vi "Goal Editor GUI.vi"(8 "error in (no error)":errorcluster, 10 "Cat Summary":refnum<class "Expense Summary.lvclass">, 11 "Database.lvclass":refnum<class "Database.lvclass">) -> (0 "error out":errorcluster, 3 "Database.lvclass":refnum<class "Database.lvclass">)   [LabVIEW 2018]
uses:
  support/classes/database/Database.lvclass
  support/classes/Expense Summary/Expense Summary.lvclass
panel:
  in  "Cancel":bool
  in  "Goal Amount":dbl
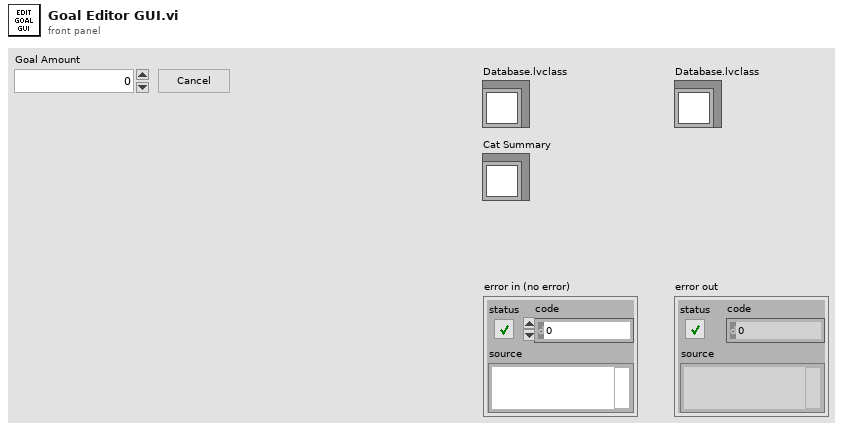
[diagram p1: front panel]
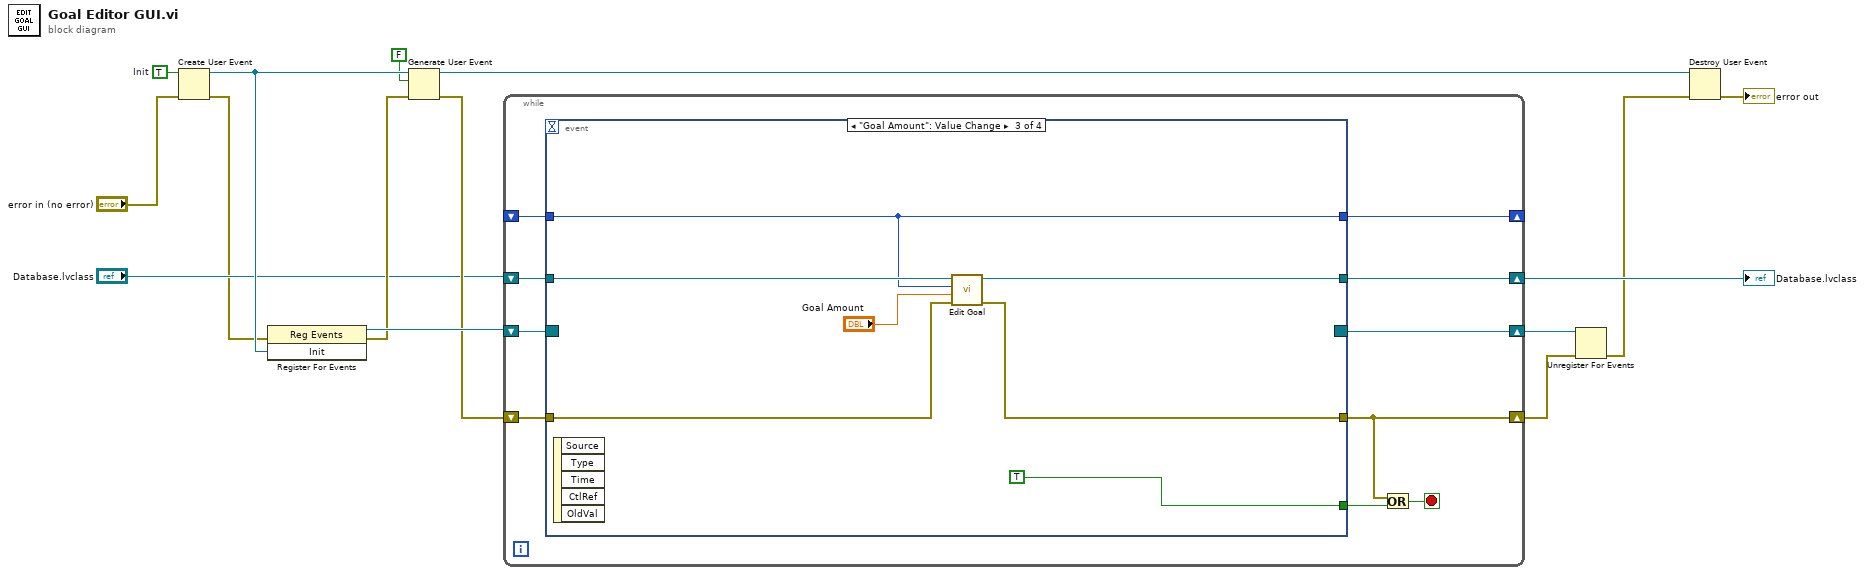
[diagram p0: block diagram]
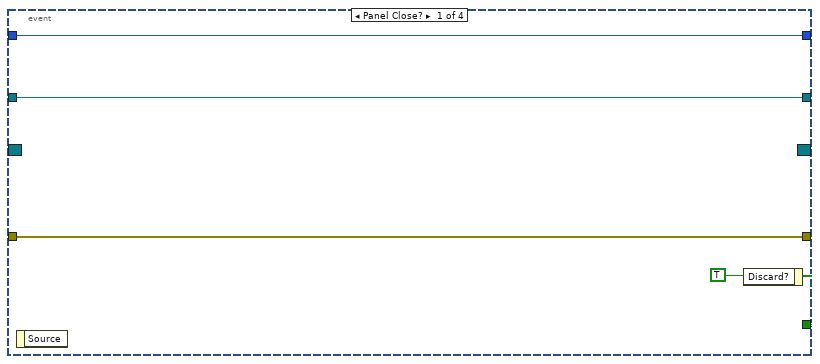
[diagram p2: hidden frame]
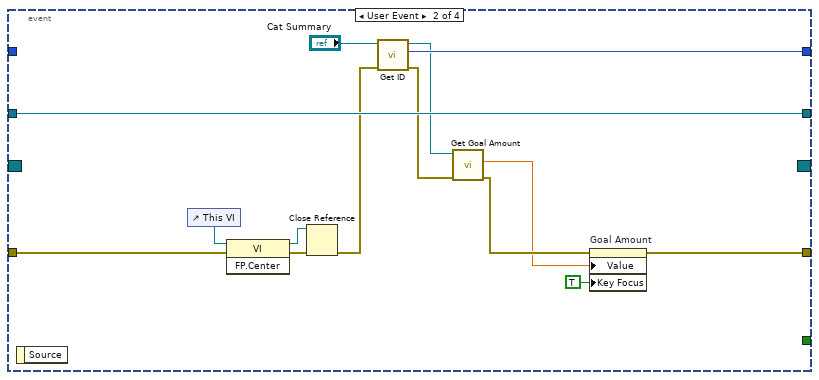
[diagram p3: hidden frame]
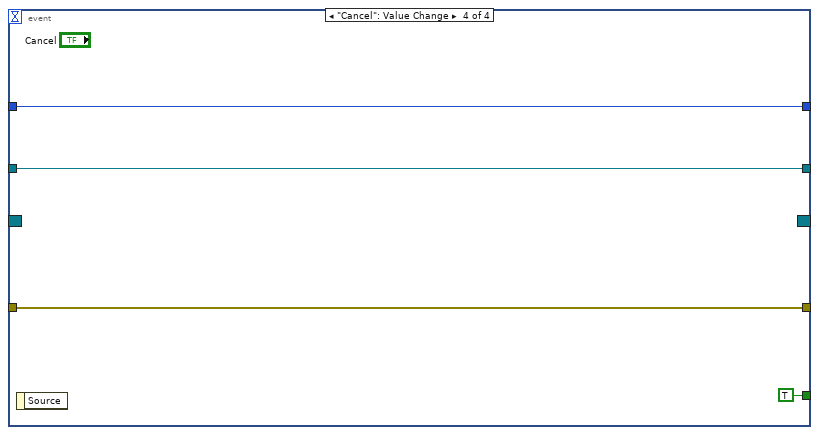
[diagram p4: hidden frame]
diagram:
  w15 = TRUE  # Init
  n1 = Create User Event(user event datatype=w15, error in="error in (no error)") -> (user event=w13:refnum<user-event>, error out=w7:errorcluster)
  n2 = register-events(error in=w7, w13) -> (reference out=w14:refnum<event-registration>, error out=w12:errorcluster)  [unwired: 1 in]
  n3 = Generate User Event(user event=w13, event data cluster=FALSE ("event data"), error in=w12) -> (user event out=w6:refnum<user-event>, error out=w11:errorcluster)  [unwired: 1 in]
  n4 = while {
    shift-right: [w23] -> w5
    shift-left: w14 -> [w25]
    shift-right: [w22] -> w4
    shift-left: w11 -> [w24]
    shift-right: [w18] -> w8
    shift-left: "Database.lvclass" -> [w19]
    shift-right: [w17] -> _
    shift-left: _ -> [w16]
    stop <- w20 stop-if-true
    n5 = event shown="[2] \"Goal Amount\": Value Change" {
      selector: w25 -> [_ _ _ _]
      dyn-events: [_ _ _ _] -> w23
      timeout: _ -> [_ _ _ _]
      tunnel: [w29 _ TRUE ("Discard?") TRUE ("Discard?")] -> w21
      tunnel: w24 -> [w28 w42 w47 w52]
      tunnel: [w28 w33 w48 w52] -> w22
      tunnel: w19 -> [w27 w39 w50 w53]
      tunnel: [w27 w39 w49 w53] -> w18
      tunnel: [w26 w37 w46 w51] -> w17
      tunnel: w16 -> [w26 _ w46 w51]
      event Panel Close? {
        w29 = TRUE ("Discard?")
        n6 = event-data() -> ()  [unwired: 1 in, 1 out]
        n7 = event-data("Discard?"=w29) -> ()  [unwired: 1 in, 1 out]
      }
      event User Event {
        n8 = event-data() -> ()  [unwired: 1 in, 1 out]
        n9 = control-ref of="This VI"() -> (w43:refnum<vi>)
        n10 = invoke class="VI" method="FP.Center"(reference=w43, error in=w42) -> (reference out=w40:refnum<vi>, error out=w41:errorcluster)  [unwired: 1 in, 1 out]
        n11 = Close Reference(reference=w40, error in (no error)=w41) -> (error out=w36:errorcluster)
        n12 = call "Get ID.vi"("error in (no error)"=w36, "Expense Summary in"="Cat Summary") -> ("error out"=w31:errorcluster, "goal_id"=w37:i32, "Expense Summary out"=w35:refnum<class "Expense Summary.lvclass">)  [unwired: 7 in]
        n13 = call "Get Goal Amount.vi"("error in (no error)"=w31, "Expense Summary in"=w35) -> ("error out"=w34:errorcluster, "Goal Amount"=w32:dbl)  [unwired: 7 in, 1 out]
        n14 = property on="Goal Amount" class="DigNum (strict)"(error in=w34, "Value"=w32, "Key Focus"=TRUE) -> (error out=w33:errorcluster)  [unwired: 1 in, 1 out]
      }
      event "Goal Amount": Value Change {
        n15 = event-data() -> ()  [unwired: 1 in, 5 out]
        n16 = call "Edit Goal.vi"("error in (no error)"=w47, "Amount"="Goal Amount", "Goal ID"=w46, "Database in"=w50) -> ("error out"=w48:errorcluster, "Database out"=w49:refnum<class "Database.lvclass">)  [unwired: 6 in]
      }
      event "Cancel": Value Change {
        n17 = event-data() -> ()  [unwired: 1 in, 1 out]
      }
    }
    n18 = Or(x=w22, y=w21) -> (x .or. y?=w20:bool)
  }
  "Database.lvclass" <- w8
  n19 = Unregister For Events(event registration refnum=w5, error in=w4) -> (error out=w2:errorcluster)
  n20 = Destroy User Event(user event=w6, error in=w2) -> (error out=→"error out":errorcluster)
